vi "QueryServer_GetRequest_Query.vi"(0 "gRPCid":T1, 3 "error in (no error)":errorcluster) -> (7 "gRPCid out":T1, 9 "query":string, 10 "error out":errorcluster)   [LabVIEW 2019, in "labview-grpc-query-server.lvlib"]
uses:
  labview-grpc-query-server.lvlib
  QueryServer_gRPCid.ctl
  QueryServer_QueryRequest.ctl
  build/Debug/labview_grpc_server.dll
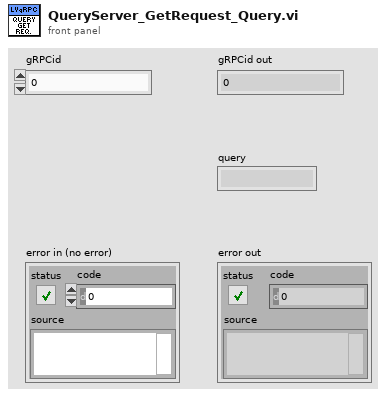
[diagram p1: front panel]
types:
  T1 = typedef "labview-grpc-query-server.lvlib/QueryServer_gRPCid.ctl" = u64
  T2 = typedef "labview-grpc-query-server.lvlib/QueryServer_QueryRequest.ctl" = cluster{"query":string}
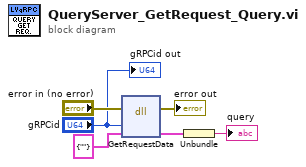
[diagram p0: block diagram]
diagram:
  n1 = dll-call lib="C:/dev/labview-grpc-server/build/Debug/labview_grpc_server.dll" fn="GetRequestData"(error in="error in (no error)", "id"="gRPCid", "data"=T2 {"query"=""} ("QueryRequest")) -> (error out=→"error out":errorcluster, "data"=w2:T2)  [unwired: 4 in, 1 out]
  n2 = Unbundle(w2) -> ("query"=→"query":string)
  "gRPCid out" <- "gRPCid"
